vi "Test - Log Status.vi"(10 "Event Data String (-)":string="Data String", 11 "Event String":string="Status String") -> (0 "error out":errorcluster)   [LabVIEW 2014]
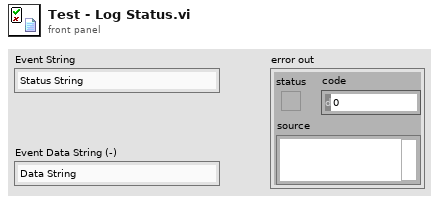
[diagram p1: front panel]
types:
  T1 = enum16{"open", "replace", "create", "open or create", "replace or create", "replace or create with confirmation"}
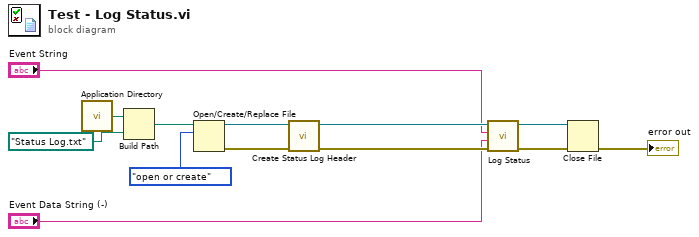
[diagram p0: block diagram]
diagram:
  n1 = call <vilib>:"Application Directory.vi"() -> ("Application Directory"=w7:path)
  n2 = Build Path(base path=w7, name or relative path=path "Status Log.txt") -> (appended path=w11:path)
  n3 = Open/Create/Replace File(file path (use dialog)=w11, operation (0:open)=T1."open or create") -> (refnum out=w8:refnum<file>, error out=w9:errorcluster)  [unwired: 4 in, 1 out]
  n4 = call "Create Status Log Header.vi"("error in"=w9, "Log File Refnum in"=w8) -> ("error out"=w13:errorcluster, "Log File Refnum out"=w12:refnum<file>)  [unwired: 8 in]
  n5 = call "Log Status.vi"("error in"=w13, "Event Data String (-)"="Event Data String (-)", "Event String"="Event String", "Log File Refnum In"=w12) -> ("error out"=w3:errorcluster, "Log File Refnum Out"=w1:refnum<file>)  [unwired: 6 in]
  n6 = Close File(refnum=w1, error in=w3) -> (error out=→"error out":errorcluster)  [unwired: 1 out]
